vi "manual_control.vi"(9 "LEFT":bool, 10 "RIGHT":bool, 11 "UP":bool) -> (3 "Array":dbl[](array[numeric]))   [LabVIEW 2016]
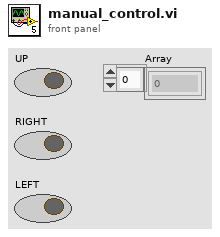
[diagram p1: front panel]
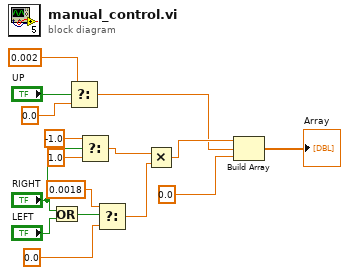
[diagram p0: block diagram]
diagram:
  n1 = Or(x="RIGHT", y="LEFT") -> (x .or. y?=w7:bool)
  n2 = Select(t=0.002, s="UP", f=0.0) -> (s? t:f=w15:dbl)
  n3 = Select(t=-1.0, s="RIGHT", f=1.0) -> (s? t:f=w14:dbl)
  n4 = Select(t=0.0018, s=w7, f=0.0) -> (s? t:f=w13:dbl)
  n5 = Multiply(x=w14, y=w13) -> (x*y=w16:dbl)
  n6 = Build Array(w16, w15, 0.0 ("element")) -> (→"Array":dbl[])
